vi "SCOPE_SetSettings.vi"(5 "Reference Point (50.0)":dbl=50.0 format="%_3f", 6 "Vertical Scale (0.005)":dbl=0.005 format="%^.3e", 7 "Time Scale (100.0e-6)":dbl=0.0001 format="%^.3e", 8 "error in (no error)":errorcluster, 10 "Configuration Cluster":T1={"General"={"Config.ini"=path "", "Default Logging Path"=path ""}, "Hardware"={"Global T VAR"="", "Global B VAR"="", "VISAS"={"GEN COM"="", "SCOPE COM"="", "VNA COM"=""}, "Connected?"={"SCOPE"=FALSE, "GEN"=FALSE, "VNA"=FALSE}}, "Operation"={"Operation Mode"=enum."Idle-Off", "Status"="", "NewLog?"=FALSE, "OvenWarn"=FALSE, "Scope Settings"={"TimeBase"=0.0, "VerticalScale"=4.0, "Channel"=enum."Channel 2"}, "Gen Settings"={"Amplitude"=0.0, "Frequency"=0.0, "Offset"=0.0}}}) -> (0 "error out":errorcluster, 2 "Configuration Cluster Out":T1={"General"={"Config.ini"=path "", "Default Logging Path"=path ""}, "Hardware"={"Global T VAR"="", "Global B VAR"="", "VISAS"={"GEN COM"="", "SCOPE COM"="", "VNA COM"=""}, "Connected?"={"SCOPE"=FALSE, "GEN"=FALSE, "VNA"=FALSE}}, "Operation"={"Operation Mode"=enum."Idle-Off", "Status"="", "NewLog?"=FALSE, "OvenWarn"=FALSE, "Scope Settings"={"TimeBase"=0.0, "VerticalScale"=4.0, "Channel"=enum."Channel 2"}, "Gen Settings"={"Amplitude"=0.0, "Frequency"=0.0, "Offset"=0.0}}})   [LabVIEW 2021]
uses:
  Config_Cluster.ctl
  Mode_Enum.ctl
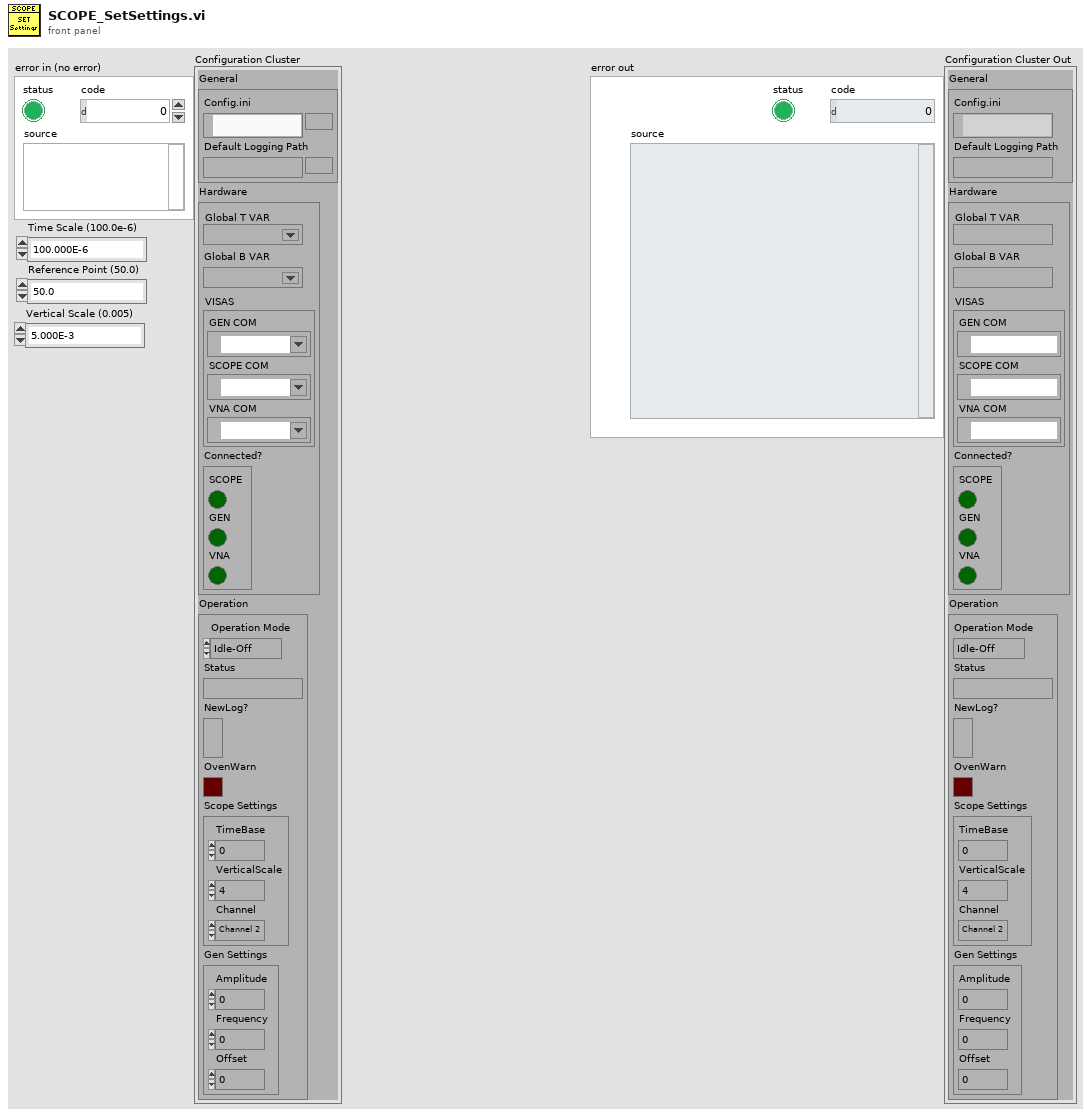
[diagram p1: front panel]
types:
  T1 = typedef "Config_Cluster.ctl" = cluster{"General":cluster{"Config.ini":path, "Default Logging Path":path}, "Hardware":cluster{"Global T VAR":refnum<k21>, "Global B VAR":refnum<k21>, "VISAS":cluster{"GEN COM":refnum<visa-resource-name>, "SCOPE COM":refnum<visa-resource-name>, "VNA COM":refnum<visa-resource-name>}, "Connected?":cluster{"SCOPE":bool, "GEN":bool, "VNA":bool}}, "Operation":cluster{"Operation Mode":T2, "Status":string, "NewLog?":bool, "OvenWarn":bool, "Scope Settings":cluster{"TimeBase":dbl, "VerticalScale":dbl, "Channel":enum16{"Channel 2", "Channel 1"}}, "Gen Settings":cluster{"Amplitude":dbl, "Frequency":dbl, "Offset":dbl}}}
  T2 = typedef "Mode_Enum.ctl" = enum16{"Logging", "Idle-Off", "Idle"}
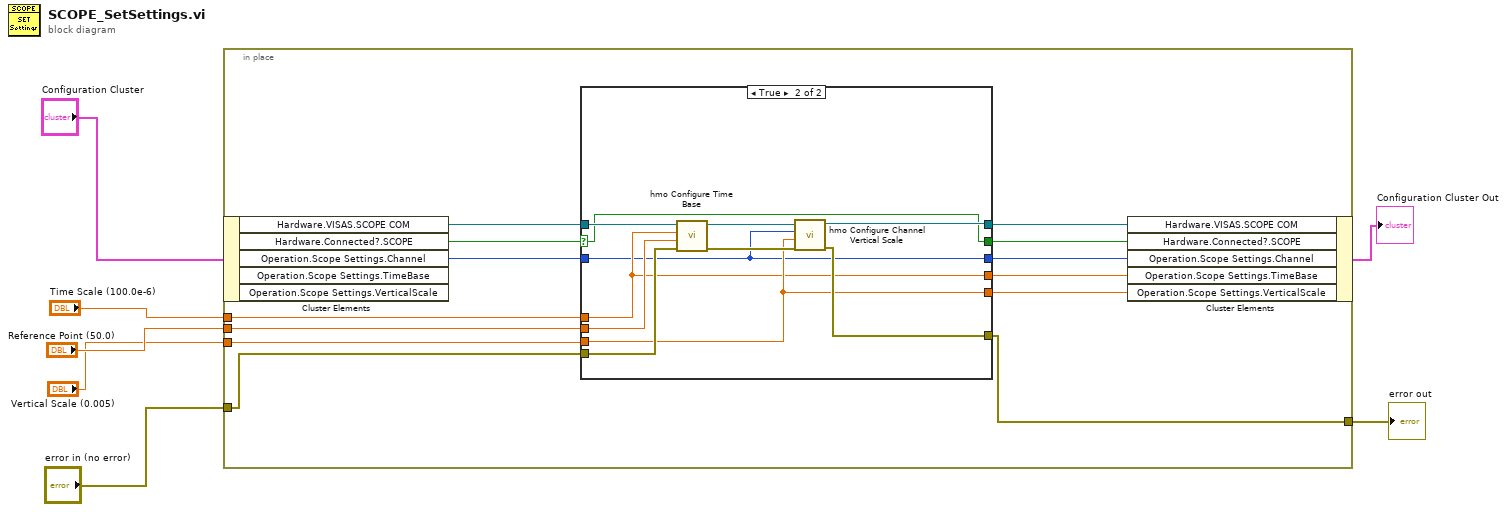
[diagram p0: block diagram]
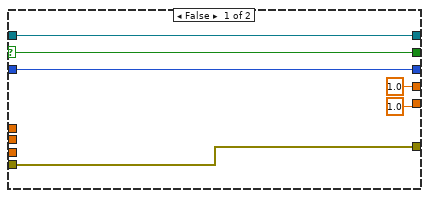
[diagram p2: hidden frame]
diagram:
  n1 = in-place {
    in-place-border: "error in (no error)" -> [w17]
    in-place-border: [w16] -> w4
    in-place-border: "Time Scale (100.0e-6)" -> [w10]
    in-place-border: "Reference Point (50.0)" -> [w9]
    in-place-border: "Vertical Scale (0.005)" -> [w8]
    n2 = in-place-cluster #1("Configuration Cluster") -> ("Hardware.VISAS.SCOPE COM"=w19:refnum<visa-resource-name>, "Hardware.Connected?.SCOPE"=w20:bool, "Operation.Scope Settings.Channel"=w14:enum16{"Channel 2", "Channel 1"})  [unwired: 2 out]
    n3 = case shown="True" w20 {
      selector: w20 -> [w26 w27]
      tunnel: w19 -> [w24 w37]
      tunnel: [w26 w27] -> w18
      tunnel: w17 -> [w25 w33]
      tunnel: [w25 w31] -> w16
      tunnel: [w24 w35] -> w15
      tunnel: w14 -> [w21 w28]
      tunnel: [w21 w28] -> w13
      tunnel: [1.0 ("Response Value") w29] -> w12
      tunnel: [1.0 ("Response Value") w30] -> w11
      tunnel: w10 -> [_ w29]
      tunnel: w9 -> [_ w34]
      tunnel: w8 -> [_ w30]
      frame False {
      }
      frame True {
        n4 = call <instrlib>:"hmo Configure Time Base.vi"("error in (no error)"=w33, "Reference Point (50.0)"=w34, "Time Scale (100.0e-6)"=w29, "VISA resource name"=w37) -> ("error out"=w32:errorcluster, "VISA resource name out"=w36:refnum<visa-resource-name>)  [unwired: 6 in]
        n5 = call <instrlib>:"hmo Configure Channel Vertical Scale.vi"("error in (no error)"=w32, "Vertical Scale (0.005)"=w30, "Channel (1)"=w28, "VISA resource name"=w36) -> ("error out"=w31:errorcluster, "VISA resource name out"=w35:refnum<visa-resource-name>)  [unwired: 6 in]
      }
    }
    n6 = in-place-cluster #1("Hardware.VISAS.SCOPE COM"=w15, "Hardware.Connected?.SCOPE"=w18, "Operation.Scope Settings.Channel"=w13, "Operation.Scope Settings.TimeBase"=w12, "Operation.Scope Settings.VerticalScale"=w11) -> (→"Configuration Cluster Out":T1)
  }
  "error out" <- w4
